vi "Application Settings Updated.vi"(8 "error in":errorcluster, 10 "Reply Payload":T1={"Settings"={"Log File Base Path"=path "", "Meta Data"={"Operator"="", "Job Number"="", "Part Number"=""}, "DAQ Settings"={"physical channel"="cDAQ9181-1913300Mod1/ai0", "minimum value"=0.0, "maximum value"=94400.0, "number of samples"=10, "rate"=125.0, "custom scale name"="Pressure"}}, "error"={"status"=FALSE, "code"=0, "source"=""}}) -> (0 "error out":errorcluster)   [LabVIEW 2025, in "Settings Editor.lvlib"]
doc: "Request Settings Editor to return the latest settings. The Settings Editor can send the applications settings as a reply or via broadcast.\n_____\nCreated using DQMH Event Scripter 4.1.0.75.\n_____\nBased on DQMH Dev Tools: Project Template 7.1.0.1503."
uses:
  Settings Editor.lvlib
  Update Application Settings (Reply Payload)--cluster.ctl
  Settings--cluster.ctl
  Test Meta Data.ctl
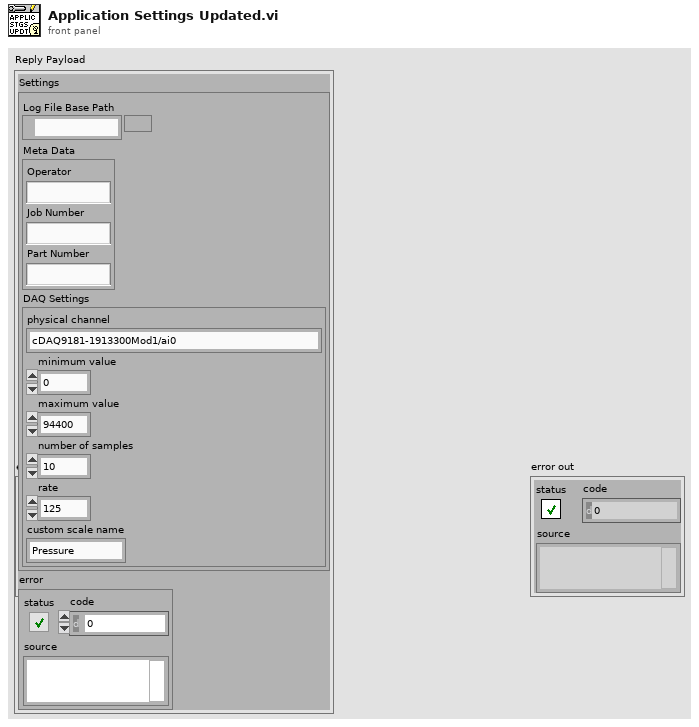
[diagram p1: front panel]
types:
  T1 = typedef "Settings Editor.lvlib/Update Application Settings (Reply Payload)--cluster.ctl" = cluster{"Settings":T2, "error":errorcluster}
  T2 = typedef "Settings Editor.lvlib/Settings--cluster.ctl" = cluster{"Log File Base Path":path, "Meta Data":T3, "DAQ Settings":cluster{"physical channel":string, "minimum value":dbl, "maximum value":dbl, "number of samples":i32, "rate":dbl, "custom scale name":string}}
  T3 = typedef "Settings Editor.lvlib/Test Meta Data.ctl" = cluster{"Operator":string, "Job Number":string, "Part Number":string}
  T4 = typedef "Settings Editor.lvlib/Broadcast Events--cluster.ctl" = cluster{"Module Did Init":refnum<user-event>, "Status Updated":refnum<user-event>, "Error Reported":refnum<user-event>, "Module Did Stop":refnum<user-event>, "Update Module Execution Status":refnum<user-event>, "Application Settings Updated":refnum<user-event>}
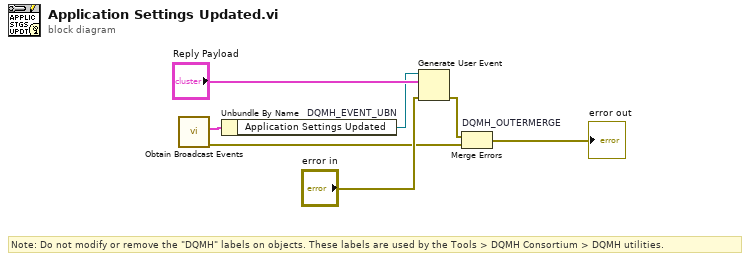
[diagram p0: block diagram]
diagram:
  # "Note: Do not modify or remove the \"DQMH\" labels on objects. These labels are used by the Tools > DQMH Consortium > DQMH utilities."
  n1 = call "Obtain Broadcast Events.vi"() -> ("error out"=w2:errorcluster, "Settings Editor Broadcast Events"=w1:T4)  [unwired: 10 in]
  n2 = Unbundle By Name "DQMH_EVENT_UBN"(w1) -> ("Application Settings Updated"=w4:refnum<user-event>)
  n3 = Generate User Event(user event=w4, event data cluster="Reply Payload", error in="error in") -> (error out=w3:errorcluster)  [unwired: 1 in, 1 out]
  n4 = Merge Errors "DQMH_OUTERMERGE"(w3, w2) -> (→"error out":errorcluster)
